vi "ADI_IMU_ADIS16470_Open.vi"(5 "Calibrate On Open":bool=TRUE, 8 "error in":errorcluster) -> (0 "error out":errorcluster, 3 "ADI IMU DevRef Out":T1)   [LabVIEW 2018, in "ADIS16470_IMU.lvlib"]
doc: "Initiates communication between an Analog Devices MXP IMU and the RoboRIO."
uses:
  ADIS16470_IMU.lvlib
  ADI_IMU_ADIS16470_IMUDevRef.ctl
  <vilib>/Rock Robotics/SystemInterfaces/spilib/spi_bus.ctl
  <vilib>/Rock Robotics/WPI/SPI/WPI_SPIMode.ctl
  <vilib>/Rock Robotics/SystemInterfaces/DIO/FPGA_DIOChannel.ctl
  <vilib>/Rock Robotics/SystemInterfaces/NetworkCommunication/NetComm_UsageReport_ResourceType.ctl
  ADI_IMU_ADIS16470_Registers.ctl
  <vilib>/Utility/error.llb/DialogType.ctl
  <vilib>/Rock Robotics/WPI/Counter/WPI_CounterDigitalInputToDigitalSource.vi
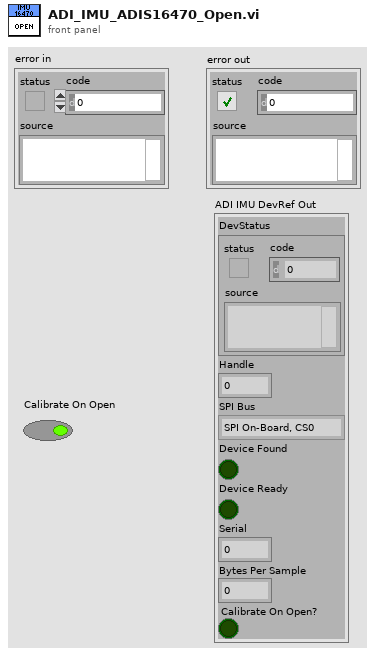
[diagram p1: front panel]
types:
  T1 = typedef "ADIS16470_IMU.lvlib/ADI_IMU_ADIS16470_IMUDevRef.ctl" = cluster{"DevStatus":errorcluster, "Handle":i32, "SPI Bus":T2, "Device Found":bool, "Device Ready":bool, "Serial":u16, "Bytes Per Sample":u16, "Calibrate On Open?":bool}
  T2 = typedef "spi_bus.ctl" = enum16{"SPI On-Board, CS0", "SPI On-Board, CS1", "SPI On-Board, CS2", "SPI On-Board, CS3", "SPI MXP", "Invalid"}
  T3 = typedef "FPGA_DIOChannel.ctl" = enum8{"DIO 0", "DIO 1", "DIO 2", "DIO 3", "DIO 4", "DIO 5", "DIO 6", "DIO 7", "DIO 8", "DIO 9", "DIO MXP 0", "DIO MXP 1", "DIO MXP 2", "DIO MXP 3", "DIO MXP 4", "DIO MXP 5", "DIO MXP 6", "DIO MXP 7", "DIO MXP 8", "DIO MXP 9", "DIO MXP 10", "DIO MXP 11", "DIO MXP 12", "DIO MXP 13", "DIO MXP 14", "DIO MXP 15", "SPI Port CS1", "SPI Port CS2", "SPI Port CS3", "SPI Port MISO", "SPI Port MOSI", "Invalid"}
  T4 = typedef "WPI_SPIMode.ctl" = enum16{"Mode 0 (Clk Idle Low,Sample on Leading)", "Mode 1 (Clk Idle Low,Sample on Trailing)", "Mode 2 (Clk Idle High,Sample on Leading)", "Mode 3 (Clk Idle High,Sample on Trailing)"}
  T5 = typedef "NetComm_UsageReport_ResourceType.ctl" = enum8{"Controller", "Module", "Language", "CANPlugin", "Accelerometer", "ADXL345", "AnalogChannel", "AnalogTrigger", "AnalogTriggerOutput", "CANJaguar", "Compressor", "Counter", "Dashboard", "DigitalInput", "DigitalOutput", "DriverStationCIO", "DriverStationEIO", "DriverStationLCD", "Encoder", "GearTooth", "Gyro", "I2C", "Framework", "Jaguar", "Joystick", "Kinect", "KinectStick", "PIDController", "Preferences", "PWM", "Relay", "RobotDrive", "SerialPort", "Servo", "Solenoid", "SPI", "Task", "Ultrasonic", "Victor", "Button", "Command", "AxisCamera", "PCVideoServer", "SmartDashboard", "Talon", "HiTechnicColorSensor", "HiTechnicAccel", "HiTechnicCompass", "SRF08", "AnalogOutput", "Victor SP", "Talon SRX", "CAN Talon SRX", "ADXL362 Accel", "ADXRS450 Gyro", "Rev SPARK", "Mindsensors SD540", "Digital Filter", "ADIS16448", "PDP", "PCM", "PigeonIMU", "Nidec Brushless", "CTRE CANifier", "CTRE Future 0", "CTRE Future 1", "CTRE Future 2", "CTRE Future 3", "CTRE Future 4", "CTRE Future 5", "CTRE Future 6", "Linear Filter", "Xbox Controller", "USB Camera", "NavX", "Pixy", "Pixy2", "ScanseSweep", "Shuffleboard", "CAN", "Digilent DMC60", "PWM Victor SPX", "Rev SPARK MAX PWM", "Rev SPARK MAX CAN", "ADIS16470"}
  T6 = typedef "ADIS16470_IMU.lvlib/ADI_IMU_ADIS16470_Registers.ctl" = u8
  T7 = typedef "WPI_DigitalOutputDevRef.ctl" = cluster{"DIO Channel":T3, "DevStatus":errorcluster}
  T8 = typedef "WPI_DigitalInputDevRef.ctl" = cluster{"DevStatus":errorcluster, "DIO Channel":T3}
  T9 = typedef "WPI_SPIDevRef.ctl" = cluster{"DevStatus":errorcluster, "Handle":i32, "SPI Bus":T2}
  T10 = typedef "FPGA_CounterEncoderSourceConvertionLVSourceType.ctl" = cluster{"DevStatus":errorcluster, "AnalogTriggerMode?":bool, "DigitalMode":cluster{"DIO Channel":T11}, "AnalogTriggerMode":cluster{"AnalogTriggerIndex":T12, "OutputType":T13}}
  T11 = typedef "FPGA_DIODigitalSourceChannel.ctl" = enum8{"DIO 0", "DIO 1", "DIO 2", "DIO 3", "DIO 4", "DIO 5", "DIO 6", "DIO 7", "DIO 8", "DIO 9", "DIO MXP 0", "DIO MXP 1", "DIO MXP 2", "DIO MXP 3", "DIO MXP 4", "DIO MXP 5", "DIO MXP 6", "DIO MXP 7", "DIO MXP 8", "DIO MXP 9", "DIO MXP 10", "DIO MXP 11", "DIO MXP 12", "DIO MXP 13", "DIO MXP 14", "DIO MXP 15", "SPI Port CS1", "SPI Port CS2", "SPI Port CS3", "SPI Port MISO", "SPI Port MOSI", "Disabled"}
  T12 = typedef "FPGA_AnalogTriggerIndex.ctl" = enum8{"Trig 0", "Trig 1", "Trig 2", "Trig 3", "Trig 4", "Trig 5", "Trig 6", "Trig 7", "Invalid"}
  T13 = typedef "FPGA_AnalogTriggerOutType.ctl" = enum16{"InWindow", "TriggerState", "Rising", "Falling"}
  T14 = typedef "DialogType.ctl" = u16
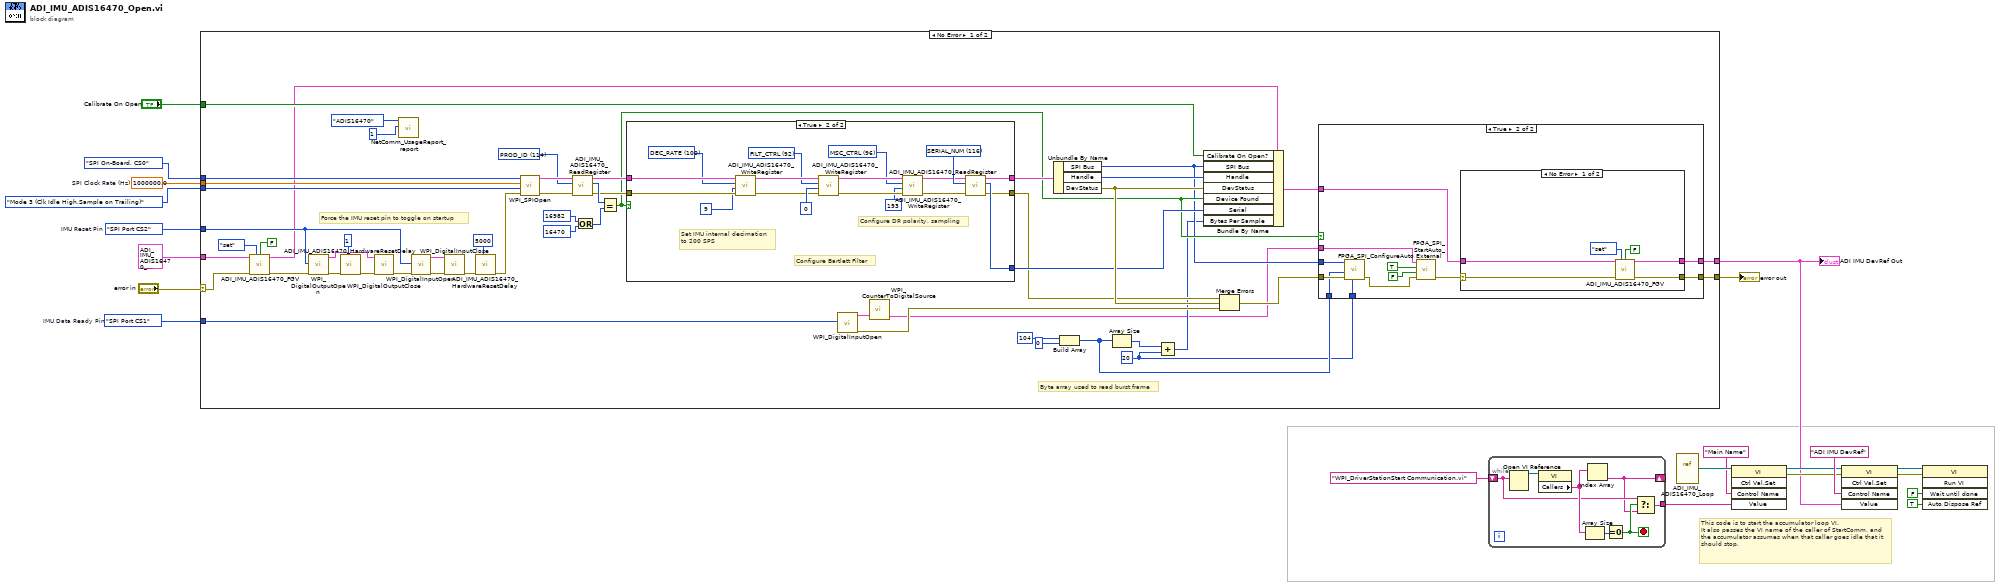
[diagram p0: block diagram]
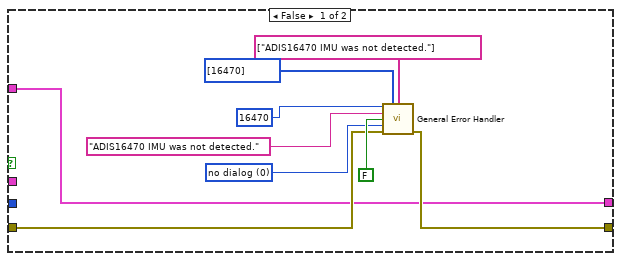
[diagram p2: hidden frame]
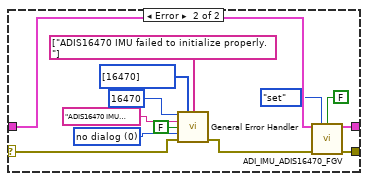
[diagram p3: hidden frame]
diagram:
  w1 = FPGA_DIOChannel."SPI Port CS1"  # IMU Data Ready Pin
  w18 = FPGA_DIOChannel."SPI Port CS2"  # IMU Reset Pin
  w21 = 1000000.0  # SPI Clock Rate (Hz)
  # "This code is to start the accumulator loop VI.\nIt also passes the VI name of the caller of StartComm, and the accumulator assumes when that caller goes idle that it should stop."
  n1 = case shown="No Error" "error in" {
    selector: "error in" -> [w33 w136]
    tunnel: w21 -> [w74 _]
    tunnel: WPI_SPIMode."Mode 3 (Clk Idle High,Sample on Trailing)" ("Mode (3)") -> [w73 _]
    tunnel: spi_bus."SPI On-Board, CS0" ("SPI Chip Select") -> [w72 _]
    tunnel: w18 -> [w71 _]
    tunnel: "Calibrate On Open" -> [w37 _]
    tunnel: [w28 w136] -> w4
    tunnel: T1 {"DevStatus"={"status"=FALSE, "code"=0, "source"=""}, "Handle"=0, "SPI Bus"=enum."SPI On-Board, CS0", "Device Found"=FALSE, "Device Ready"=FALSE, "Serial"=0, "Bytes Per Sample"=0, "Calibrate On Open?"=FALSE} ("SimpleGyroDevRef 2") -> [w31 w135]
    tunnel: [w27 w135] -> w2
    tunnel: w1 -> [w26 _]
    frame No Error {
      w25 = T6 114 items=["DIAG_STAT"=2, "X_GYRO"=6, "Y_GYRO"=10, "Z_GYRO"=14, "X_ACCEL"=18, "Y_ACCEL"=22, "Z_ACCEL"=26, "TEMP_OUT"=28, "TIME_STAMP"=30, "DATA_CNTR"=34, "FILT_CTRL"=92, "MSC_CTRL"=96, "DEC_RATE"=100, "NULL_CFG"=102, "GLOB_CMD"=104, "PROD_ID"=114, "SERIAL_NUM"=116] ("ADIS16470 Register")
      w39 = 20 ("dimension size")
      # "Byte array used to read burst frame"
      # "Force the IMU reset pin to toggle on startup"
      n2 = call "ADI_IMU_ADIS16470_FGV.vi"("ADI IMU DevRef"=w31, "Operation"=enum16{"set", "get", "set reset"}."set", "Sensor Ready?"=FALSE, "error in"=w33) -> ("ADI IMU DevRef Out"=w30:T1, "error out"=w32:errorcluster)  [unwired: 6 in, 4 out]
      n3 = call <vilib>:"WPI_DigitalOutputOpen.vi"("error in (no error)"=w32, "DIO Channel"=w71) -> ("error out"=w52:errorcluster, "DigitalOutputDevRef"=w46:T7)  [unwired: 8 in]
      n4 = call "ADI_IMU_ADIS16470_HardwareResetDelay.vi"("Delay (ms)"=u32 1, "error in"=w52) -> ("error out"=w53:errorcluster)  [unwired: 9 in]
      n5 = call <vilib>:"WPI_DigitalOutputClose.vi"("error in (no error)"=w53, "DigitalOutputDevRef"=w46) -> ("error out"=w51:errorcluster)  [unwired: 9 in]
      n6 = call <vilib>:"NetComm_UsageReport_report.vi"("Instance Number"=u8 1, "Resource Type"=NetComm_UsageReport_ResourceType."ADIS16470") -> ()  [unwired: 10 in]
      n7 = call <vilib>:"WPI_DigitalInputOpen.vi"("error in (no error)"=w51, "DIO Channel"=w71) -> ("error out"=w50:errorcluster, "DigitalInputDevRef"=w49:T8)  [unwired: 8 in]
      n8 = call <vilib>:"WPI_DigitalInputClose.vi"("error in (no error)"=w50, "DigitalInputDevRef"=w49) -> ("error out"=w48:errorcluster)  [unwired: 9 in]
      n9 = call "ADI_IMU_ADIS16470_HardwareResetDelay.vi"("Delay (ms)"=u32 5000, "error in"=w48) -> ("error out"=w67:errorcluster)  [unwired: 9 in]
      n10 = call <vilib>:"WPI_SPIOpen.vi"("error in"=w67, "Mode (3)"=w73, "Clock Rate (Hz)"=w74, "SPI Bus"=w72) -> ("error out"=w63:errorcluster, "SPIDevRef"=w64:T9)  [unwired: 6 in]
      n11 = call "ADI_IMU_ADIS16470_ReadRegister.vi"("error in (no error)"=w63, "ADIS16448 Register"=w25, "SPIDevRef in"=w64) -> ("error out"=w60:errorcluster, "Register Value"=w62:u16, "SPIDevRef out"=w61:T9)  [unwired: 6 in]
      n12 = Or(x=u16 16982 ("y"), y=u16 16470) -> (x .or. y?=w22:u16)
      n13 = Equal?(x=w62, y=w22) -> (x = y?=w56:bool)
      n14 = case shown="True" w56 {
        tunnel: [_ w133] -> w68
        tunnel: [w116 w118] -> w59
        tunnel: [w115 w117] -> w58
        tunnel: w61 -> [w116 w128]
        tunnel: w60 -> [w115 w127]
        frame False {
        }
        frame True {
          w121 = T6 116 items=["DIAG_STAT"=2, "X_GYRO"=6, "Y_GYRO"=10, "Z_GYRO"=14, "X_ACCEL"=18, "Y_ACCEL"=22, "Z_ACCEL"=26, "TEMP_OUT"=28, "TIME_STAMP"=30, "DATA_CNTR"=34, "FILT_CTRL"=92, "MSC_CTRL"=96, "DEC_RATE"=100, "NULL_CFG"=102, "GLOB_CMD"=104, "PROD_ID"=114, "SERIAL_NUM"=116] ("ADIS16470 Register")
          w122 = T6 96 items=["DIAG_STAT"=2, "X_GYRO"=6, "Y_GYRO"=10, "Z_GYRO"=14, "X_ACCEL"=18, "Y_ACCEL"=22, "Z_ACCEL"=26, "TEMP_OUT"=28, "TIME_STAMP"=30, "DATA_CNTR"=34, "FILT_CTRL"=92, "MSC_CTRL"=96, "DEC_RATE"=100, "NULL_CFG"=102, "GLOB_CMD"=104, "PROD_ID"=114, "SERIAL_NUM"=116] ("ADIS16470 Register")
          w123 = T6 92 items=["DIAG_STAT"=2, "X_GYRO"=6, "Y_GYRO"=10, "Z_GYRO"=14, "X_ACCEL"=18, "Y_ACCEL"=22, "Z_ACCEL"=26, "TEMP_OUT"=28, "TIME_STAMP"=30, "DATA_CNTR"=34, "FILT_CTRL"=92, "MSC_CTRL"=96, "DEC_RATE"=100, "NULL_CFG"=102, "GLOB_CMD"=104, "PROD_ID"=114, "SERIAL_NUM"=116] ("ADIS16470 Register")
          w124 = T6 100 items=["DIAG_STAT"=2, "X_GYRO"=6, "Y_GYRO"=10, "Z_GYRO"=14, "X_ACCEL"=18, "Y_ACCEL"=22, "Z_ACCEL"=26, "TEMP_OUT"=28, "TIME_STAMP"=30, "DATA_CNTR"=34, "FILT_CTRL"=92, "MSC_CTRL"=96, "DEC_RATE"=100, "NULL_CFG"=102, "GLOB_CMD"=104, "PROD_ID"=114, "SERIAL_NUM"=116] ("ADIS16470 Register")
          # "Configure DR polarity, sampling"
          # "Configure Bartlett Filter"
          # "Set IMU internal decimation\nto 200 SPS"
          n15 = call "ADI_IMU_ADIS16470_WriteRegister.vi"("error in (no error)"=w127, "Data"=u16 9, "Register"=w124, "SPIDevRef in"=w128) -> ("error out"=w131:errorcluster, "SPIDevRef out"=w132:T9)  [unwired: 6 in]
          n16 = call "ADI_IMU_ADIS16470_WriteRegister.vi"("error in (no error)"=w131, "Data"=u16 0, "Register"=w123, "SPIDevRef in"=w132) -> ("error out"=w129:errorcluster, "SPIDevRef out"=w130:T9)  [unwired: 6 in]
          n17 = call "ADI_IMU_ADIS16470_WriteRegister.vi"("error in (no error)"=w129, "Data"=u16 193, "Register"=w122, "SPIDevRef in"=w130) -> ("error out"=w119:errorcluster, "SPIDevRef out"=w120:T9)  [unwired: 6 in]
          n18 = call "ADI_IMU_ADIS16470_ReadRegister.vi"("error in (no error)"=w119, "ADIS16448 Register"=w121, "SPIDevRef in"=w120) -> ("error out"=w117:errorcluster, "Register Value"=w133:u16, "SPIDevRef out"=w118:T9)  [unwired: 6 in]
        }
      }
      n19 = call <vilib>:"WPI_DigitalInputOpen.vi"("DIO Channel"=w26) -> ("error out"=w45:errorcluster, "DigitalInputDevRef"=w38:T8)  [unwired: 9 in]
      n20 = call-poly <vilib>:"WPI_CounterToDigitalSource.vi"("DigitalInputDevRef"=w38) -> ("Digital Source"=w36:T10)  [unwired: 6 in]
      n21 = Unbundle By Name(w59) -> ("SPI Bus"=w55:T2, "Handle"=w70:i32, "DevStatus"=w69:errorcluster)
      n22 = Build Array(u8 104 ("hi"), u8 0 ("element")) -> (w42:u8[])
      n23 = Array Size(array=w42) -> (size(s)=w41:i32)
      n24 = Add(x=w41, y=w39) -> (x+y=w40:i32)
      n25 = Bundle By Name(cluster=w30, "Calibrate On Open?"=w37, "SPI Bus"=w55, "Handle"=w70, "DevStatus"=w69, "Device Found"=w56, "Serial"=w68, "Bytes Per Sample"=w40) -> (w29:T1)
      n26 = Merge Errors(w58, w69, w45) -> (w57:errorcluster)
      n27 = case shown="True" w56 {
        tunnel: w57 -> [w77 w95]
        tunnel: w55 -> [_ w94]
        tunnel: w42 -> [_ w91]
        tunnel: w39 -> [_ w90]
        tunnel: w36 -> [_ w89]
        tunnel: w29 -> [w75 w86]
        tunnel: [w76 w85] -> w28
        tunnel: [w75 w84] -> w27
        frame False {
          w80 = T14 0 items=["no dialog", "OK message", "continue or stop message", "OK message + warnings", "continue/stop + warnings"] ("type of dialog (OK msg:1)")
          n28 = call <vilib>:"General Error Handler.vi"("[error code] (0)"=16470, "[user-defined codes]"=i32[] [16470], "[user-defined descriptions]"=string[] ["ADIS16470 IMU was not detected."], "[error source] (\" \")"="ADIS16470 IMU was not detected." ("[error source] (\" \")"), "search ni.com link visible?(T)"=FALSE, "type of dialog (OK msg:1)"=w80, "error in (no error)"=w77) -> ("error out"=w76:errorcluster)  [unwired: 4 in, 4 out]
        }
        frame True {
          n29 = call <vilib>:"FPGA_SPI_ConfigureAuto.vi"("SPI Auto Zero Byte Count"=w90, "error in"=w95, "SPI Auto TX Byte Array"=w91, "SPI Bus"=w94) -> ("error out"=w88:errorcluster)  [unwired: 7 in]
          n30 = call <vilib>:"FPGA_SPI_StartAuto_External.vi"("error in (no error)"=w88, "Falling Edge"=FALSE, "Rising Edge"=TRUE, "Source"=w89) -> ("error out"=w87:errorcluster)  [unwired: 7 in]
          n31 = case shown="No Error" w87 {
            selector: w87 -> [w98 w108]
            tunnel: w86 -> [w99 w105]
            tunnel: [w97 w106] -> w85
            tunnel: [w96 w107] -> w84
            frame No Error {
              n32 = call "ADI_IMU_ADIS16470_FGV.vi"("ADI IMU DevRef"=w99, "Operation"=enum16{"set", "get", "set reset"}."set", "Sensor Ready?"=FALSE, "error in"=w98) -> ("ADI IMU DevRef Out"=w96:T1, "error out"=w97:errorcluster)  [unwired: 6 in, 4 out]
            }
            frame Error {
              w111 = T14 0 items=["no dialog", "OK message", "continue or stop message", "OK message + warnings", "continue/stop + warnings"] ("type of dialog (OK msg:1)")
              n33 = call <vilib>:"General Error Handler.vi"("[error code] (0)"=16470, "[user-defined codes]"=i32[] [16470], "[user-defined descriptions]"=string[] ["ADIS16470 IMU failed to initialize properly."], "[error source] (\" \")"="ADIS16470 IMU failed to initialize properly. IMU was not properly initialized." ("[error source] (\" \")"), "search ni.com link visible?(T)"=FALSE, "type of dialog (OK msg:1)"=w111, "error in (no error)"=w108) -> ("error out"=w104:errorcluster)  [unwired: 4 in, 4 out]
              n34 = call "ADI_IMU_ADIS16470_FGV.vi"("ADI IMU DevRef"=w105, "Operation"=enum16{"set", "get", "set reset"}."set", "Sensor Ready?"=FALSE, "error in"=w104) -> ("ADI IMU DevRef Out"=w107:T1, "error out"=w106:errorcluster)  [unwired: 6 in, 4 out]
            }
          }
        }
      }
    }
    frame Error {
    }
  }
  "error out" <- w4
  "ADI IMU DevRef Out" <- w2
  n35 = while {
    shift-right: [w138] -> _
    shift-left: "WPI_DriverStationStart Communication.vi" -> [w139]
    tunnel: [w137] -> w8
    stop <- w140 stop-if-true
    n36 = Open VI Reference(vi path=w139) -> (vi reference=w143:refnum<vi>)  [unwired: 1 in, 5 out]
    n37 = property class="VI"(reference=w143) -> ("Callers"=w141:string[])  [unwired: 1 in, 2 out]
    n38 = Array Size(array=w141) -> (size(s)=w142:i32)
    n39 = Index Array(array=w141) -> (element=w138:string)  [unwired: 1 in]
    n40 = Equal To 0?(x=w142) -> (x = 0?=w140:bool)
    n41 = Select(t=w139, s=w140, f=w138) -> (s? t:f=w137:string)
  }
  n42 = vi-ref "ADI_IMU_ADIS16470_Loop.vi"() -> (w10:refnum<vi>)
  n43 = invoke class="VI" method="Ctrl Val.Set"(reference=w10, "Control Name"="Main Name", "Value"=w8) -> (reference out=w7:refnum<vi>, error out=w12:errorcluster)  [unwired: 2 in, 3 out]
  n44 = invoke class="VI" method="Ctrl Val.Set"(reference=w7, error in=w12, "Control Name"="ADI IMU DevRef", "Value"=w2) -> (reference out=w17:refnum<vi>, error out=w13:errorcluster)  [unwired: 1 in, 3 out]
  n45 = invoke class="VI" method="Run VI"(reference=w17, error in=w13, "Wait until done"=FALSE ("Wait Until Done"), "Auto Dispose Ref"=TRUE ("Auto Dispose Reference")) -> ()  [unwired: 1 in, 5 out]
